vi "FPGA_Digital.vi"() -> ()   [LabVIEW 2021]
uses:
  <vilib>/rvi/interface/RandomDataEmulation/niFpgaRandomDataHandleErrors.vi
  <vilib>/rvi/eio/common/nirviEmuTemplateMethod_errors.vi
  <vilib>/rvi/DataTransferAndStorage/Container/XNode/niFpgaContainer.xnode
  <vilib>/rvi/interface/RandomDataEmulation/nirviRandomDataFpgaReadWriteTemplate.vi
  <vilib>/eio/EIONode/EIONode.xnode
panel:
  in  "Number_of_Steps":i32=3
  in  "Wait_time(uSec)":u32
  out "Numeric":i16
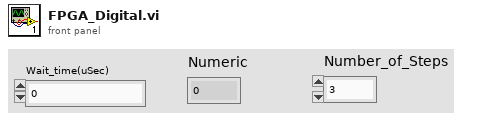
[diagram p1: front panel]
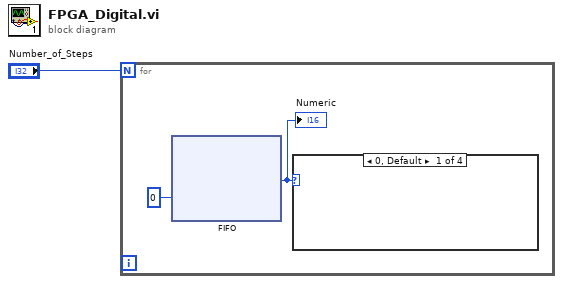
[diagram p0: block diagram]
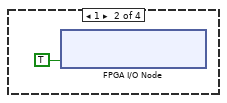
[diagram p2: hidden frame]
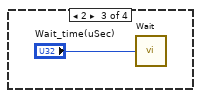
[diagram p3: hidden frame]
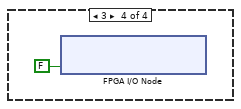
[diagram p4: hidden frame]
diagram:
  n1 = for {
    N: "Number_of_Steps" -> [_]
    n2 = xnode "FIFO"("Timeout"=0) -> ("Element"=w2:i16)  [unwired: 1 in, 2 out]
    "Numeric" <- w2
    n3 = case shown="0, Default" w2 {
      frame 0, Default {
      }
      frame 1 {
        n4 = xnode "FPGA I/O Node"("Connector0/DIO0"=TRUE) -> ()  [unwired: 1 in, 1 out]
      }
      frame 2 {
        n5 = call "Wait"("Count(uSec)"="Wait_time(uSec)") -> ()  [unwired: 1 out]
      }
      frame 3 {
        n6 = xnode "FPGA I/O Node"("Connector0/DIO0"=FALSE) -> ()  [unwired: 1 in, 1 out]
      }
    }
  }
